vi "Turbulence_3.0_LevelProbe.vi"() -> ()   [LabVIEW 2018]
uses:
  Quantum Composers 9000 Series.lvlib
  LightField Automation.lvclass
  Mercury iXX.lvlib
  Temperature (Read).vi
  Temperature.lvlib
  Open Temperature Device.vi
  Comms Transport Layer.ctl
  Keithley 2600 Series.lvlib
  Channel.ctl
  Open System.vi
  System.lvlib
  Catalogue (Read).vi
panel:
  out "time string":string
  out "Timestamp":string
  out "Log Error":errorcluster
  in  "CLOSE":bool
  in  "RECORD":bool
  in  "Turbulence":T1(tab)
  in  "BIN":u16(ring) items=["1x1", "2x2", "4x4"]
  in  "MODE":u16(ring) items=["Normal", "DIF"]
  in  "Enable":bool
  out "Rate (Hz)":dbl
  out "Neutron Counts":dbl
  in  "Script\nEnd":u32=1 step=1
  in  "Sample Space Pump":bool
  in  "Siphon Pump":bool
  in  "Neutron Shutter":bool
  in  "Manual Script Entry (0)":string
  in  "READY":bool
  out "Power (mW)":dbl format="%_3f"
  out "Tank Pressure 2 (Torr)":string="0.0"
  in  "LIGHTFIELD":bool
  in  "SCRIPTING":bool
  out "Liquid He Level":dbl(slide) min=0.0 max=100.0 step=0.01 scale=0.0..50.0 scale format="%#_2f"
  in  "Top Coil":bool
  in  "Number of Frames":i32=500 min=0 step=1
  in  "On CCD Accumulations":i32=3 min=0 step=1
  out "Tank Pressure 1 (Torr)":string="0.0"
  out "Cell Temp (K)":dbl
  in  "Data folder":path=path "C:/Data"
  out "Cryostat Temp (K)":dbl
  in  "Data Interval (s)":dbl=1.0 min=0.4 max=10.0 step=0.05
  in  "RUN/STOP":bool
  in  "Bottom Coil":bool
  in  "Bottom Coil (mA)":dbl min=-1000.0 max=1000.0 step=1e-05
  in  "Top Coil (mA)":dbl min=-1000.0 max=1000.0 step=1e-05
  in  "Percent Open":i32 min=0 max=100 step=5
  out "Liquid Level":dbl format="%_2f"
  in  "COOLDOWN":bool
  in  "Script\n#":u32=1 step=1
  in  "Kill Switch":bool
  in  "DATA":bool
  out "Scripting \nError":T2
  in  "Shutter Mode":u16(ring) items=["Manual"=1, "XGate"=5]
  in  "Log Pressure":bool
  out "4He Pressure (Torr)":string="-0.1"
  out "3He Pressure (Torr)":string="1"
  out "Temperature Error":errorcluster={"status"=TRUE, "code"=-1073807339, "source"="VISA Read in Mercury iXX.lvlib:Query (Dynamic).vit->Mercury iXX.lvlib:Query (Low Level).vi:10049->Mercury iXX.lvlib:Query.vi:3960048->Mercury iXX.lvlib:Read (Str).vi:5300004->Mercury iXX.lvlib:System.lvlib:Catalogue (Read).vi->Turbulence.vi"}
  out "File I/O Error":errorcluster
  out "4He Gauge Error":errorcluster={"status"=TRUE, "code"=-1073807343, "source"="VISA Open in Turbulence.vi"}
  out "Heater Error":errorcluster={"status"=FALSE, "code"=1073676293, "source"="VISA Read in Keithley 2600 Series.lvlib:Print Number.vi->Keithley 2600 Series.lvlib:Measure.vi->Turbulence.vi"}
  out "Pulse Generator Error":errorcluster
  out "3He Gauge Error":errorcluster={"status"=FALSE, "code"=1073676293, "source"="VISA Read in 3HeClose.vi->Turbulence.vi"}
  out "Relay Errror":errorcluster
  out "Zaber Motor Error":errorcluster
  out "Level Probe Error":errorcluster={"status"=TRUE, "code"=56, "source"="TCP Read in Command.vi->Turbulence.vi"}
  out "LightField Error":errorcluster
  # "Camera Controls"
  # "Temperature Readout"
  # "Pressure Readout"
  # "Liquid He Level"
  # "Automation"
  # "Heater Controls"
  # "Relay Controls"
  # "Needle Valve Control"
  # "Neutron Shutter"
  # "Optical Shutter"
  # "Siphon Pump"
  # "Laser Power Meter"
  # "Sample Space\nPump"
  # "Quartz\nCell"
  # "4"
  # "3psi relief"
  # "4L Tank"
  # "Turbo Pump"
  # "3"
  # "10psi relief"
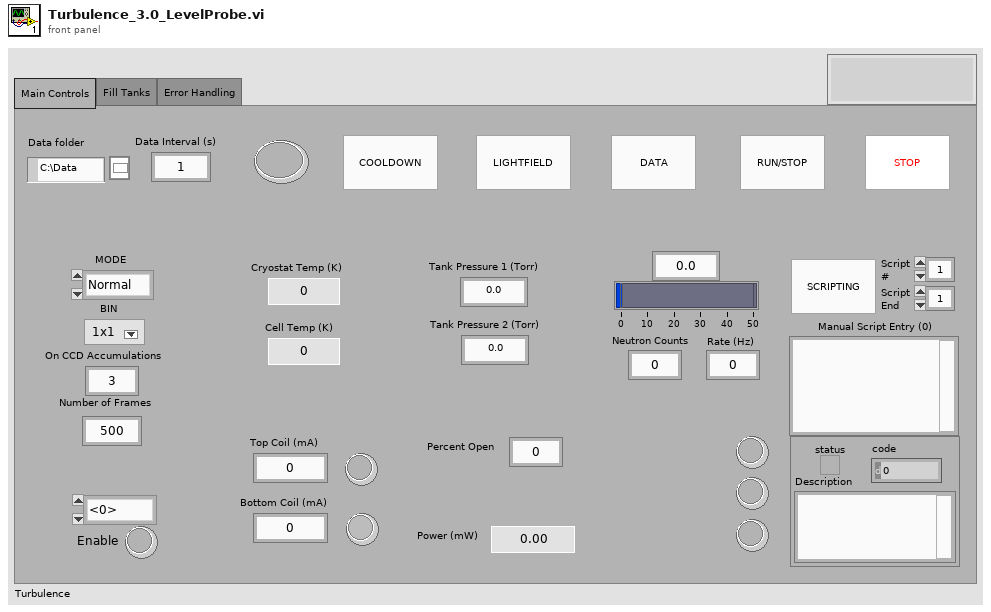
[diagram p1: front panel]
types:
  T1 = enum32{"Main Controls", "Fill Tanks", "Error Handling"}
  T2 = cluster{"status":bool, "code":i32, "Description":string}
  T3 = typedef "Mercury iXX.lvlib/Comms Transport Layer.ctl" = enum16{"Ethernet TCP/IP", "USB", "ISOBus - RS-232", "GPIB"}
  T4 = typedef "Mercury iXX.lvlib/Mercury Reference.ctl" = cluster{"Comms":refnum<visa-resource-name>, "Device ID":string[], "Comms Layer":T3, "Command":string, "Query reference":T5}
  T5 = typedef "Mercury iXX.lvlib/Query Dynamic Reference.ctl" = refnum<vi>
  T6 = enum32{"Current", "Voltage", "IV", "Resistance", "Power"}
  T7 = typedef "Keithley 2600 Series.lvlib/Channel.ctl" = enum32{"Channel A", "Channel B"}
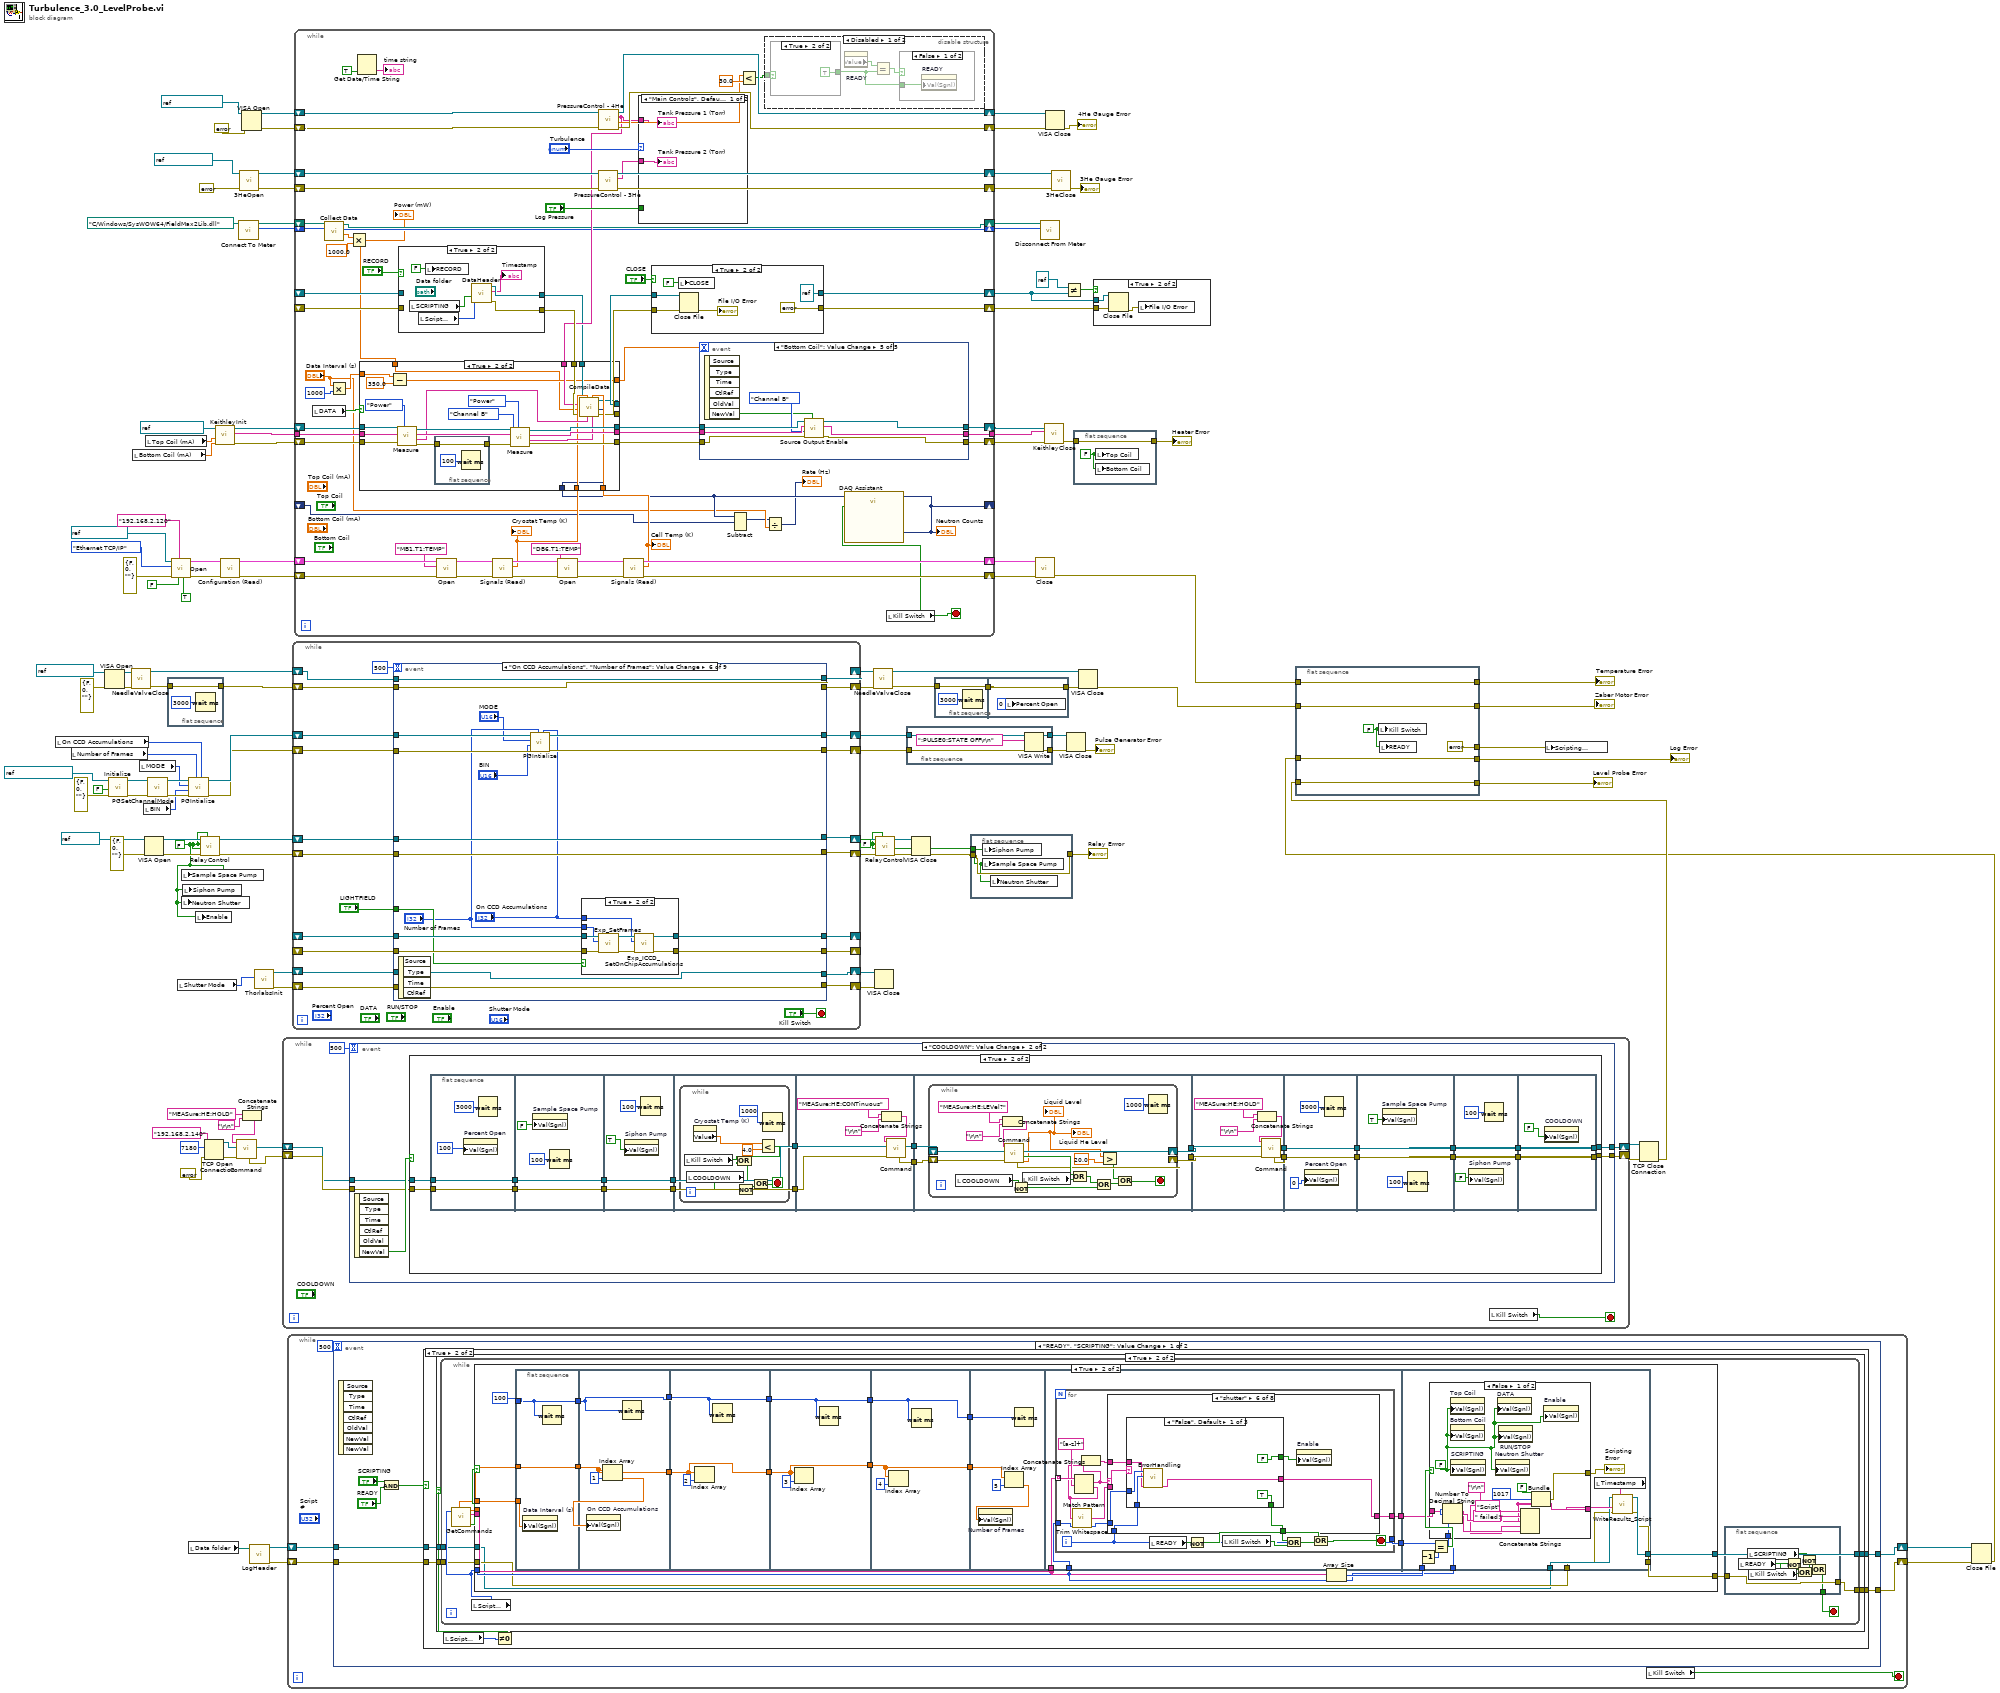
[diagram p0: block diagram]
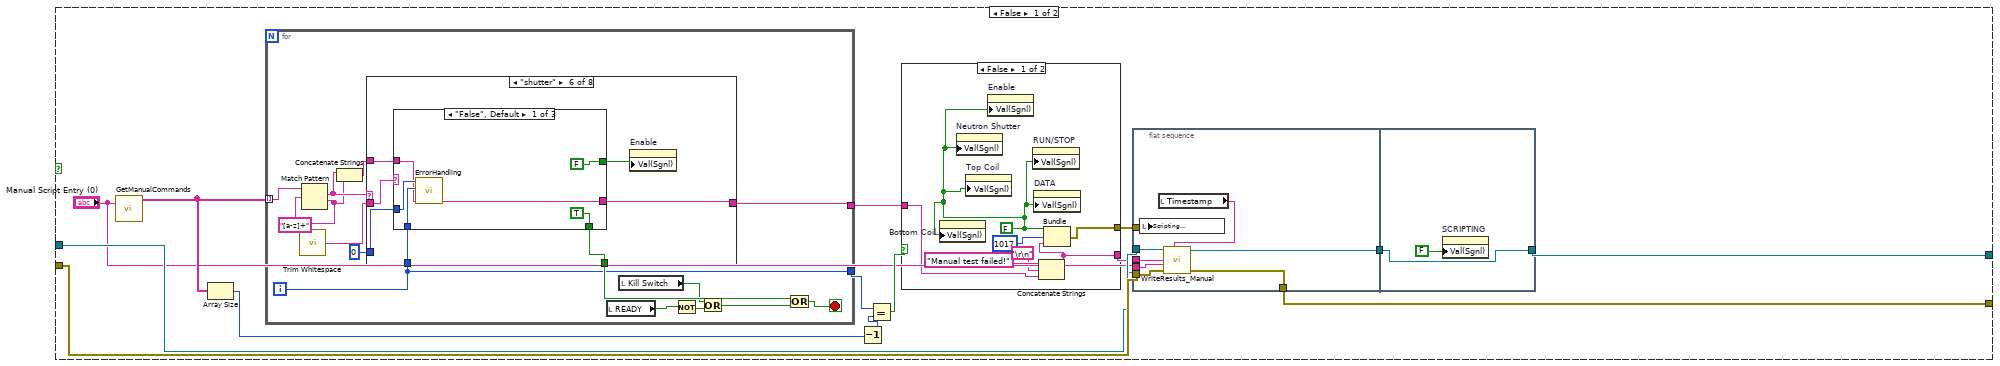
[diagram p3: hidden frame]
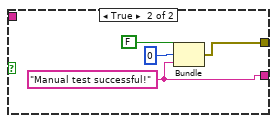
[diagram p4: hidden frame]
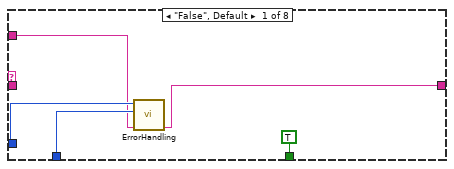
[diagram p5: hidden frame]
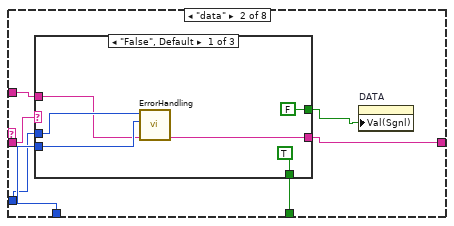
[diagram p6: hidden frame]
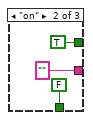
[diagram p7: hidden frame]
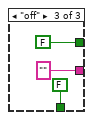
[diagram p8: hidden frame]
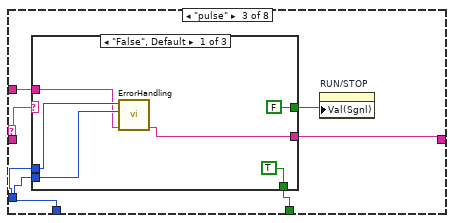
[diagram p9: hidden frame]
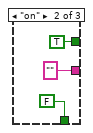
[diagram p10: hidden frame]
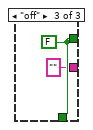
[diagram p11: hidden frame]
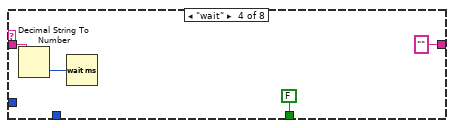
[diagram p12: hidden frame]
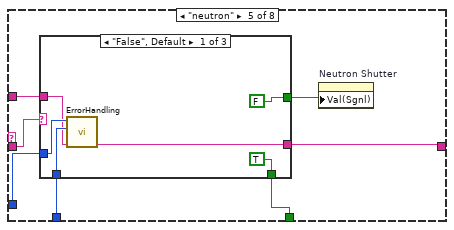
[diagram p13: hidden frame]
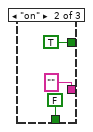
[diagram p14: hidden frame]
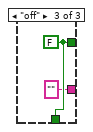
[diagram p15: hidden frame]
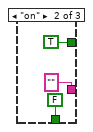
[diagram p16: hidden frame]
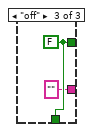
[diagram p17: hidden frame]
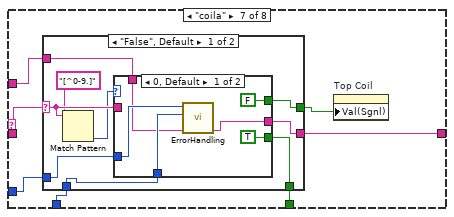
[diagram p18: hidden frame]
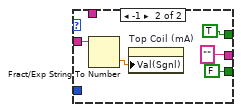
[diagram p19: hidden frame]
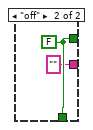
[diagram p20: hidden frame]
diagram:
  w33 = FALSE ("Siphon Pump")
  w17 = FALSE ("Siphon Pump")
  n1 = local read "On CCD Accumulations"() -> (w4:i32)
  n2 = local read "Number of Frames"() -> (w3:i32)
  n3 = VISA Open(error in (no error)=errorcluster {"status"=FALSE, "code"=0, "source"=""}, VISA resource name=refnum<visa-resource-name> "ZaberMotor") -> (VISA resource name=w10:refnum<visa-resource-name>, error out=w11:errorcluster)  [unwired: 3 in]
  n4 = call "Initialize.vi"("error in (no error)"=errorcluster {"status"=FALSE, "code"=0, "source"=""}, "Reset? (T: Yes)"=FALSE, "VISA resource name"=refnum<visa-resource-name> "PulseGenerator" ("Pulse generater (COM3)")) -> ("error out"=w24:errorcluster, "VISA resource name out"=w22:refnum<visa-resource-name>)  [unwired: 7 in]
  n5 = call "NeedleValveClose.vi"("error in (no error)"=w11, "VISA resource name"=w10) -> ("error out"=w12:errorcluster, "VISA resource name out"=w55:refnum<visa-resource-name>)  [unwired: 8 in]
  n6 = local read "Bottom Coil (mA)"() -> (w69:dbl)
  n7 = local read "MODE"() -> (w1:u16)
  n8 = local read "BIN"() -> (w2:u16)
  n9 = VISA Open(error in (no error)=errorcluster {"status"=FALSE, "code"=0, "source"=""} ("error in (no error) 2"), VISA resource name=refnum<visa-resource-name> "Relays" ("Pressure Gauge")) -> (VISA resource name=w94:refnum<visa-resource-name>, error out=w96:errorcluster)  [unwired: 3 in]
  n10 = local read "Top Coil (mA)"() -> (w70:dbl)
  n11 = call "PGSetChannelMode.vi"("error in"=w24, "VISA resource name"=w22) -> ("error out"=w23:errorcluster, "VISA resource name out"=w21:refnum<visa-resource-name>)  [unwired: 8 in]
  n12 = flat-sequence {
    tunnel: w12 -> [w123]
    tunnel: [w123] -> w56
    frame #0 {
      n13 = Wait (ms)(milliseconds to wait=u32 3000) -> ()  [unwired: 1 out]
    }
  }
  n14 = call-poly "Open.vi"("Clear Previous Connections (False)"=TRUE, "ID Query (True)"=FALSE, "IP Address"="192.168.2.120", "error in (no error)"=errorcluster {"status"=FALSE, "code"=0, "source"=""}, "Comms Layer"=Comms_Transport_Layer."Ethernet TCP/IP", "VISA resource name"=refnum<visa-resource-name> "MercuryiTC") -> ("error out"=w115:errorcluster, "Mercury Reference Out"=w116:T4)  [unwired: 1 in, 3 out]
  n15 = local read "Shutter Mode"() -> (w5:u16)
  n16 = local write "Sample Space Pump"(w17) -> ()
  n17 = local write "Neutron Shutter"(w17) -> ()
  n18 = local write "Siphon Pump"(w17) -> ()
  n19 = local read "Data folder"() -> (w31:path)
  n20 = call "PGIntialize.vi"("On CCD Accumulations"=w4, "Number of Frames"=w3, "error in"=w23, "BIN"=w2, "MODE"=w1, "VISA resource name"=w21) -> ("error out"=w120:errorcluster, "VISA resource name out"=w121:refnum<visa-resource-name>)  [unwired: 4 in]
  n21 = local write "Enable"(w17) -> ()
  n22 = call "RelayControl.vi"("Neutron Shutter"=w17, "Error In"=w96, "Sample Space Pump"=w17, "Siphon Pump"=w17, "Relay In"=w94) -> ("Error Out"=w95:errorcluster, "Relay Out"=w93:refnum<visa-resource-name>)  [unwired: 5 in]
  n23 = TCP Open Connection(address="192.168.2.140", remote port or service name=u16 7180, error in (no error)=errorcluster {"status"=FALSE, "code"=0, "source"=""}) -> (connection ID=w80:refnum<k5>, error out=w81:errorcluster)  [unwired: 2 in]
  n24 = call "KeithleyInit.vi"("Bottom Coil (mA)"=w69, "Top Coil (mA)"=w70, "KeithleyVISA In"=refnum<visa-resource-name> "Keithley2614B" ("VISA resource name")) -> ("error out"=w73:errorcluster, "Node Out"=w74:string, "KeithleyVISA Out"=w72:refnum<visa-resource-name>)  [unwired: 6 in]
  n25 = call-poly "Configuration (Read).vi"("error in"=w115, "Mercury Reference In"=w116) -> ("error out"=w111:errorcluster, "Mercury Reference Out"=w112:T4)  [unwired: 6 in, 2 out]
  n26 = call "Connect To Meter.vi"("Location of FieldMax2Lib.dll in"=path "C:/Windows/SysWOW64/FieldMax2Lib.dll") -> ("Meter ID out"=w41:i32, "Location of FieldMax2Lib.dll out"=w40:path)  [unwired: 6 in, 1 out]
  n27 = call "3HeOpen.vi"("error in (no error)"=errorcluster {"status"=FALSE, "code"=0, "source"=""} ("error in (no error) 2"), "VISA resource name"=refnum<visa-resource-name> "3HePressure" ("Pressure Gauge")) -> ("error out"=w98:errorcluster, "VISA resource name out"=w97:refnum<visa-resource-name>)  [unwired: 8 in]
  n28 = VISA Open(error in (no error)=errorcluster {"status"=FALSE, "code"=0, "source"=""} ("error in (no error) 2"), VISA resource name=refnum<visa-resource-name> "TankPressure" ("Pressure Gauge")) -> (VISA resource name=w108:refnum<visa-resource-name>, error out=w109:errorcluster)  [unwired: 3 in]
  n29 = Concatenate Strings("MEASure:HE:HOLD" ("Command"), "\r\n") -> (w82:string)
  n30 = call "Command.vi"("error in"=w81, "connection ID"=w80, "Command"=w82) -> ("connection ID 2"=w79:refnum<k5>, "error out"=w78:errorcluster)  [unwired: 3 in, 4 out]
  n31 = call "LogHeader.vi"("Data folder"=w31) -> ("error out"=w29:errorcluster, "refnum out"=w30:refnum<file>)  [unwired: 9 in]
  n32 = call "ThorlabsInit.vi"("Shutter Mode"=w5) -> ("error out"=w18:errorcluster, "VISA resource name out"=w19:refnum<visa-resource-name>)  [unwired: 9 in]
  n33 = while {
    shift-right: [w125] -> w86
    shift-left: w78 -> [w128]
    shift-right: [w126] -> w85
    shift-left: w79 -> [w127]
    stop <- w130 stop-if-true
    n34 = event shown="[1] \"COOLDOWN\": Value Change" {
      selector: _ -> [_ _]
      dyn-events: _ -> [_ _]
      timeout: 500 -> [_ _]
      tunnel: [w132 w133] -> w126
      tunnel: [w131 w134] -> w125
      tunnel: w128 -> [w131 w136]
      tunnel: w127 -> [w132 w135]
      event Timeout {
        n35 = event-data() -> ()  [unwired: 1 in, 3 out]
      }
      event "COOLDOWN": Value Change {
        n36 = event-data() -> ("NewVal"=w137:bool)  [unwired: 1 in, 5 out]
        n37 = case shown="True" w137 {
          tunnel: [w138 w157] -> w133
          tunnel: [w139 w156] -> w134
          tunnel: w136 -> [w139 w163]
          tunnel: w135 -> [w138 w161]
          frame False {
          }
          frame True {
            n38 = flat-sequence {
              tunnel: w161 -> [w166]
              tunnel: w163 -> [w167]
              tunnel: [w167] -> w149
              tunnel: [w166] -> w148
              tunnel: [w171] -> w147
              tunnel: [w170] -> w145
              tunnel: w149 -> [w171]
              tunnel: w148 -> [w170]
              tunnel: w147 -> [w175]
              tunnel: [w175] -> w146
              tunnel: w145 -> [w174]
              tunnel: [w174] -> w144
              tunnel: [w177] -> w162
              tunnel: w146 -> [w177]
              tunnel: w144 -> [w176]
              tunnel: [w176] -> w160
              tunnel: w162 -> [w190]
              tunnel: w160 -> [w189]
              tunnel: [w188] -> w159
              tunnel: [w187] -> w158
              tunnel: w159 -> [w195]
              tunnel: w158 -> [w194]
              tunnel: [w197] -> w153
              tunnel: [w196] -> w151
              tunnel: w153 -> [w219]
              tunnel: [w216] -> w152
              tunnel: w151 -> [w218]
              tunnel: [w217] -> w150
              tunnel: w152 -> [w226]
              tunnel: [w226] -> w155
              tunnel: w150 -> [w225]
              tunnel: [w225] -> w154
              tunnel: w155 -> [w230]
              tunnel: w154 -> [w229]
              tunnel: [w230] -> w143
              tunnel: [w229] -> w142
              tunnel: w143 -> [w234]
              tunnel: w142 -> [w233]
              tunnel: [w234] -> w141
              tunnel: [w233] -> w140
              tunnel: [w236] -> w156
              tunnel: [w237] -> w157
              tunnel: w141 -> [w237]
              tunnel: w140 -> [w236]
              frame #0 {
                n39 = property on="Percent Open" class="DigNum (strict)"("Val(Sgnl)"=100 ("Percent Open")) -> ()  [unwired: 2 in, 2 out]
                n40 = Wait (ms)(milliseconds to wait=u32 3000) -> ()  [unwired: 1 out]
              }
              frame #1 {
                n41 = property on="Sample Space Pump" class="Bool (strict)"("Val(Sgnl)"=FALSE ("Sample Space Pump")) -> ()  [unwired: 2 in, 2 out]
                n42 = Wait (ms)(milliseconds to wait=u32 100) -> ()  [unwired: 1 out]
              }
              frame #2 {
                n43 = property on="Siphon Pump" class="Bool (strict)"("Val(Sgnl)"=TRUE ("Siphon Pump")) -> ()  [unwired: 2 in, 2 out]
                n44 = Wait (ms)(milliseconds to wait=u32 100) -> ()  [unwired: 1 out]
              }
              frame #3 {
                n45 = while {
                  stop <- w181 stop-if-true
                  n46 = local read "Kill Switch"() -> (w184:bool)
                  n47 = local read "COOLDOWN"() -> (w179:bool)
                  n48 = property on="Cryostat Temp (K)" class="DigNum (strict)"() -> ("Value"=w186:dbl)  [unwired: 2 in, 2 out]
                  n49 = Not(x=w179) -> (.not. x?=w178:bool)
                  n50 = Less?(x=w186, y=4.0) -> (x < y?=w183:bool)
                  n51 = Or(x=w184, y=w183) -> (x .or. y?=w180:bool)
                  n52 = Or(x=w180, y=w178) -> (x .or. y?=w181:bool)
                  n53 = Wait (ms)(milliseconds to wait=u32 1000) -> ()  [unwired: 1 out]
                }
              }
              frame #4 {
                n54 = Concatenate Strings("MEASure:HE:CONTinuous" ("Command"), "\r\n") -> (w191:string)
                n55 = call "Command.vi"("error in"=w190, "connection ID"=w189, "Command"=w191) -> ("connection ID 2"=w187:refnum<k5>, "error out"=w188:errorcluster)  [unwired: 3 in, 4 out]
              }
              frame #5 {
                n56 = while {
                  shift-right: [w213] -> w197
                  shift-left: w194 -> [w214]
                  shift-right: [w207] -> w196
                  shift-left: w195 -> [w215]
                  stop <- w202 stop-if-true
                  n57 = local read "COOLDOWN"() -> (w199:bool)
                  n58 = Concatenate Strings("MEASure:HE:LEVel?" ("Command"), "\r\n") -> (w212:string)
                  n59 = call "Command.vi"("error in"=w215, "connection ID"=w214, "Command"=w212) -> ("Dbl_out"=w205:dbl, "Error"=w208:bool, "connection ID 2"=w213:refnum<k5>, "error out"=w207:errorcluster)  [unwired: 3 in, 2 out]
                  "Liquid He Level" <- w205
                  "Liquid Level" <- w205
                  n60 = Not(x=w199) -> (.not. x?=w198:bool)
                  n61 = local read "Kill Switch"() -> (w209:bool)
                  n62 = Or(x=w208, y=w209) -> (x .or. y?=w201:bool)
                  n63 = Or(x=w201, y=w198) -> (x .or. y?=w200:bool)
                  n64 = Greater?(x=w205, y=20.0) -> (0:w203:bool)
                  n65 = Or(x=w203, y=w200) -> (x .or. y?=w202:bool)
                  n66 = Wait (ms)(milliseconds to wait=u32 1000) -> ()  [unwired: 1 out]
                }
              }
              frame #6 {
                n67 = Concatenate Strings("MEASure:HE:HOLD" ("Command"), "\r\n") -> (w220:string)
                n68 = call "Command.vi"("error in"=w218, "connection ID"=w219, "Command"=w220) -> ("connection ID 2"=w216:refnum<k5>, "error out"=w217:errorcluster)  [unwired: 3 in, 4 out]
              }
              frame #7 {
                n69 = property on="Percent Open" class="DigNum (strict)"("Val(Sgnl)"=0 ("Percent Open")) -> ()  [unwired: 2 in, 2 out]
                n70 = Wait (ms)(milliseconds to wait=u32 3000) -> ()  [unwired: 1 out]
              }
              frame #8 {
                n71 = property on="Sample Space Pump" class="Bool (strict)"("Val(Sgnl)"=TRUE ("Sample Space Pump")) -> ()  [unwired: 2 in, 2 out]
                n72 = Wait (ms)(milliseconds to wait=u32 100) -> ()  [unwired: 1 out]
              }
              frame #9 {
                n73 = property on="Siphon Pump" class="Bool (strict)"("Val(Sgnl)"=FALSE ("Siphon Pump")) -> ()  [unwired: 2 in, 2 out]
                n74 = Wait (ms)(milliseconds to wait=u32 100) -> ()  [unwired: 1 out]
              }
              frame #10 {
                n75 = property on="COOLDOWN" class="Bool (strict)"("Val(Sgnl)"=FALSE ("COOLDOWN")) -> ()  [unwired: 2 in, 2 out]
              }
            }
          }
        }
      }
    }
    n76 = local read "Kill Switch"() -> (w130:bool)
  }
  n77 = while {
    shift-right: [w239] -> w28
    shift-left: w30 -> [w240]
    shift-right: [w238] -> w27
    shift-left: w29 -> [w241]
    stop <- w243 stop-if-true
    n78 = event shown="[0] \"READY\", \"SCRIPTING\": Value Change" {
      selector: _ -> [_ _]
      dyn-events: _ -> [_ _]
      timeout: 500 -> [_ _]
      tunnel: w241 -> [w247 w727]
      tunnel: w240 -> [w248 w728]
      tunnel: [w246 w728] -> w239
      tunnel: [w245 w727] -> w238
      event "READY", "SCRIPTING": Value Change {
        n79 = event-data() -> ()  [unwired: 1 in, 7 out]
        n80 = And(x="SCRIPTING", y="READY") -> (x .and. y?=w244:bool)
        n81 = case shown="True" w244 {
          tunnel: w248 -> [w252 w256]
          tunnel: w247 -> [w251 w255]
          tunnel: [w252 w253] -> w246
          tunnel: [w251 w254] -> w245
          frame False {
          }
          frame True {
            n82 = local read "Script\n#"() -> (w258:u32)
            n83 = Not Equal To 0?(x=w258) -> (x != 0?=w257:bool)
            n84 = case shown="True" w257 {
              tunnel: w256 -> [w264 w451]
              tunnel: w255 -> [w265 w452]
              tunnel: [w259 w449] -> w254
              tunnel: [w260 w450] -> w253
              frame False {
                n85 = call "GetManualCommands.vi"("Manual Script Entry (0)"="Manual Script Entry (0)") -> ("Commands"=w272:string[])  [unwired: 10 in]
                n86 = Array Size(array=w272) -> (size(s)=w268:i32)
                n87 = for {
                  tunnel: w272 -> [w307] mode=indexing
                  tunnel: [w298] -> w271
                  tunnel: [w297] -> w266
                  i -> [w298]
                  stop <- w304 stop-if-true
                  n88 = Match Pattern(string=w307, regular expression="[a-z]+") -> (match substring=w296:string, after substring=w295:string)  [unwired: 1 in, 2 out]
                  n89 = call "Trim Whitespace.vi"("string"=w295) -> ("trimmed string"=w306:string)  [unwired: 1 in]
                  n90 = Concatenate Strings(w296, w295) -> (w294:string)
                  n91 = case shown="\"shutter\"" w296 {
                    tunnel: w306 -> [_ w320 w339 w354 w361 w379 w397 w426]
                    tunnel: [TRUE ("Top Coil") w319 w336 FALSE ("Top Coil") w358 w376 w396 w425] -> w303
                    tunnel: w298 -> [w312 w318 w338 _ w360 w378 w395 w424]
                    tunnel: u32 0 ("Script Number") -> [w311 w317 w337 _ w359 w377 w394 w423]
                    tunnel: [w310 w315 w334 "" ("Error String") w356 w375 w392 w421] -> w297
                    tunnel: w294 -> [w309 w314 w333 _ w355 w374 w391 w420]
                    frame "False", Default {
                      n92 = call "ErrorHandling.vi"("Bad Command"=w309, "Line #"=w312, "Script #"=w311) -> ("Error String"=w310:string)  [unwired: 8 in]
                    }
                    frame "data" {
                      n93 = case shown="\"False\", Default" w320 {
                        tunnel: [FALSE ("DATA") TRUE ("DATA") FALSE ("DATA")] -> w316
                        tunnel: [TRUE ("Top Coil") FALSE ("Top Coil") FALSE ("Top Coil")] -> w319
                        tunnel: w318 -> [w323 _ _]
                        tunnel: w317 -> [w324 _ _]
                        tunnel: [w322 "" ("Error String") "" ("Error String")] -> w315
                        tunnel: w314 -> [w321 _ _]
                        frame "False", Default {
                          n94 = call "ErrorHandling.vi"("Bad Command"=w321, "Line #"=w323, "Script #"=w324) -> ("Error String"=w322:string)  [unwired: 8 in]
                        }
                        frame "on" {
                        }
                        frame "off" {
                        }
                      }
                      n95 = property on="DATA" class="Bool (strict)"("Val(Sgnl)"=w316) -> ()  [unwired: 2 in, 2 out]
                    }
                    frame "pulse" {
                      n96 = case shown="\"False\", Default" w339 {
                        tunnel: [FALSE ("Top Coil") TRUE ("Top Coil") w350] -> w335
                        tunnel: [TRUE FALSE w350] -> w336
                        tunnel: w338 -> [w343 _ _]
                        tunnel: w337 -> [w342 _ _]
                        tunnel: [w341 "" ""] -> w334
                        tunnel: w333 -> [w340 _ _]
                        frame "False", Default {
                          n97 = call "ErrorHandling.vi"("Bad Command"=w340, "Line #"=w343, "Script #"=w342) -> ("Error String"=w341:string)  [unwired: 8 in]
                        }
                        frame "on" {
                        }
                        frame "off" {
                          w350 = FALSE ("Top Coil")
                        }
                      }
                      n98 = property on="RUN/STOP" class="Bool (strict)"("Val(Sgnl)"=w335) -> ()  [unwired: 2 in, 2 out]
                    }
                    frame "wait" {
                      n99 = Decimal String To Number(string=w354) -> (number=w353:i32)  [unwired: 2 in, 1 out]
                      n100 = Wait (ms)(milliseconds to wait=w353) -> ()  [unwired: 1 out]
                    }
                    frame "neutron" {
                      n101 = case shown="\"False\", Default" w361 {
                        tunnel: w360 -> [w367 _ _]
                        tunnel: w359 -> [w366 _ _]
                        tunnel: [TRUE ("Top Coil") FALSE ("Top Coil") w372] -> w358
                        tunnel: [FALSE ("Neutron Shutter") TRUE ("Neutron Shutter") w372] -> w357
                        tunnel: [w363 "" ("Error String") "" ("Error String")] -> w356
                        tunnel: w355 -> [w362 _ _]
                        frame "False", Default {
                          n102 = call "ErrorHandling.vi"("Bad Command"=w362, "Line #"=w367, "Script #"=w366) -> ("Error String"=w363:string)  [unwired: 8 in]
                        }
                        frame "on" {
                        }
                        frame "off" {
                          w372 = FALSE ("Neutron Shutter")
                        }
                      }
                      n103 = property on="Neutron Shutter" class="Bool (strict)"("Val(Sgnl)"=w357) -> ()  [unwired: 2 in, 2 out]
                    }
                    frame "shutter" {
                      n104 = case shown="\"False\", Default" w379 {
                        tunnel: w378 -> [w385 _ _]
                        tunnel: w377 -> [w384 _ _]
                        tunnel: [TRUE ("Top Coil") FALSE ("Top Coil") w390] -> w376
                        tunnel: [FALSE ("Neutron Shutter") TRUE ("Neutron Shutter") w390] -> w373
                        tunnel: [w381 "" ("Error String") "" ("Error String")] -> w375
                        tunnel: w374 -> [w380 _ _]
                        frame "False", Default {
                          n105 = call "ErrorHandling.vi"("Bad Command"=w380, "Line #"=w385, "Script #"=w384) -> ("Error String"=w381:string)  [unwired: 8 in]
                        }
                        frame "on" {
                        }
                        frame "off" {
                          w390 = FALSE ("Neutron Shutter")
                        }
                      }
                      n106 = property on="Enable" class="Bool (strict)"("Val(Sgnl)"=w373) -> ()  [unwired: 2 in, 2 out]
                    }
                    frame "coila" {
                      n107 = case shown="\"False\", Default" w397 {
                        selector: w397 -> [w404 _]
                        tunnel: [w406 w419] -> w393
                        tunnel: [w405 w419] -> w396
                        tunnel: w395 -> [w401 _]
                        tunnel: w394 -> [w400 _]
                        tunnel: [w399 "" ("Error String")] -> w392
                        tunnel: w391 -> [w398 _]
                        frame "False", Default {
                          n108 = Match Pattern(string=w404, regular expression="[^0-9.]") -> (offset past match=w402:i32)  [unwired: 1 in, 3 out]
                          n109 = case shown="0, Default" w402 {
                            tunnel: [FALSE ("Top Coil") TRUE ("Top Coil")] -> w406
                            tunnel: [TRUE FALSE] -> w405
                            tunnel: w404 -> [_ w415]
                            tunnel: w401 -> [w410 _]
                            tunnel: w400 -> [w409 _]
                            tunnel: [w408 ""] -> w399
                            tunnel: w398 -> [w407 _]
                            frame 0, Default {
                              n110 = call "ErrorHandling.vi"("Bad Command"=w407, "Line #"=w410, "Script #"=w409) -> ("Error String"=w408:string)  [unwired: 8 in]
                            }
                            frame -1 {
                              n111 = Fract/Exp String To Number(string=w415) -> (number=w414:dbl)  [unwired: 3 in, 1 out]
                              n112 = property on="Top Coil (mA)" class="DigNum (strict)"("Val(Sgnl)"=w414) -> ()  [unwired: 2 in, 2 out]
                            }
                          }
                        }
                        frame "off" {
                          w419 = FALSE ("Top Coil")
                        }
                      }
                      n113 = property on="Top Coil" class="Bool (strict)"("Val(Sgnl)"=w393) -> ()  [unwired: 2 in, 2 out]
                    }
                    frame "coilb" {
                      n114 = case shown="\"False\", Default" w426 {
                        selector: w426 -> [w433 _]
                        tunnel: [w432 w448] -> w422
                        tunnel: [w431 w448] -> w425
                        tunnel: w424 -> [w430 _]
                        tunnel: w423 -> [w429 _]
                        tunnel: [w428 ""] -> w421
                        tunnel: w420 -> [w427 _]
                        frame "False", Default {
                          n115 = Match Pattern(string=w433, regular expression="[^0-9.]") -> (offset past match=w434:i32)  [unwired: 1 in, 3 out]
                          n116 = case shown="0, Default" w434 {
                            tunnel: w433 -> [_ w446]
                            tunnel: [FALSE TRUE] -> w432
                            tunnel: [TRUE FALSE] -> w431
                            tunnel: w430 -> [w439 _]
                            tunnel: w429 -> [w438 _]
                            tunnel: [w437 ""] -> w428
                            tunnel: w427 -> [w436 _]
                            frame 0, Default {
                              n117 = call "ErrorHandling.vi"("Bad Command"=w436, "Line #"=w439, "Script #"=w438) -> ("Error String"=w437:string)  [unwired: 8 in]
                            }
                            frame -1 {
                              n118 = Fract/Exp String To Number(string=w446) -> (number=w443:dbl)  [unwired: 3 in, 1 out]
                              n119 = property on="Bottom Coil (mA)" class="DigNum (strict)"("Val(Sgnl)"=w443) -> ()  [unwired: 2 in, 2 out]
                            }
                          }
                        }
                        frame "off" {
                          w448 = FALSE
                        }
                      }
                      n120 = property on="Bottom Coil" class="Bool (strict)"("Val(Sgnl)"=w422) -> ()  [unwired: 2 in, 2 out]
                    }
                  }
                  n121 = local read "READY"() -> (w299:bool)
                  n122 = local read "Kill Switch"() -> (w300:bool)
                  n123 = Not(x=w299) -> (.not. x?=w302:bool)
                  n124 = Or(x=w300, y=w302) -> (x .or. y?=w301:bool)
                  n125 = Or(x=w303, y=w301) -> (x .or. y?=w304:bool)
                }
                n126 = Decrement(x=w268) -> (x-1=w270:i32)
                n127 = Equal?(x=w271, y=w270) -> (x = y?=w269:bool)
                n128 = case shown="False" w269 {
                  tunnel: [w288 w291] -> w267
                  tunnel: w266 -> [w286 _]
                  tunnel: [w284 w290] -> w262
                  frame False {
                    w283 = FALSE ("status")
                    n129 = property on="Bottom Coil" class="Bool (strict)"("Val(Sgnl)"=w283) -> ()  [unwired: 2 in, 2 out]
                    n130 = property on="Neutron Shutter" class="Bool (strict)"("Val(Sgnl)"=w283) -> ()  [unwired: 2 in, 2 out]
                    n131 = property on="Top Coil" class="Bool (strict)"("Val(Sgnl)"=w283) -> ()  [unwired: 2 in, 2 out]
                    n132 = property on="Enable" class="Bool (strict)"("Val(Sgnl)"=w283) -> ()  [unwired: 2 in, 2 out]
                    n133 = property on="RUN/STOP" class="Bool (strict)"("Val(Sgnl)"=w283) -> ()  [unwired: 2 in, 2 out]
                    n134 = property on="DATA" class="Bool (strict)"("Val(Sgnl)"=w283) -> ()  [unwired: 2 in, 2 out]
                    n135 = Concatenate Strings("Manual test failed!" ("Description"), "\r\n", w286) -> (w284:string)
                    n136 = Bundle("status"=w283, "code"=1017, w284) -> (w288:cluster{"status":bool, "code":i32, string})  [unwired: 1 in]
                  }
                  frame True {
                    w290 = "Manual test successful!" ("Description")
                    n137 = Bundle("status"=FALSE, "code"=0, "Description"=w290) -> (w291:T2)  [unwired: 1 in]
                  }
                }
                n138 = flat-sequence {
                  tunnel: w267 -> [w280]
                  tunnel: w265 -> [w276]
                  tunnel: w264 -> [w279]
                  tunnel: "Manual Script Entry (0)" -> [w278]
                  tunnel: w262 -> [w277]
                  tunnel: [w275] -> w261
                  tunnel: [w274] -> w259
                  tunnel: w261 -> [w282]
                  tunnel: [w282] -> w260
                  frame #0 {
                    n139 = local write "Scripting \nError"(w280) -> ()
                    n140 = local read "Timestamp"() -> (w273:string)
                    n141 = call "WriteResults_Manual.vi"("Timestamp"=w273, "error in"=w276, "Result"=w277, "Commands"=w278, "refnum in"=w279) -> ("error out"=w274:errorcluster, "refnum out"=w275:refnum<file>)  [unwired: 5 in]
                  }
                  frame #1 {
                    n142 = property on="SCRIPTING" class="Bool (strict)"("Val(Sgnl)"=FALSE ("Value (Signaling)")) -> ()  [unwired: 2 in, 2 out]
                  }
                }
              }
              frame True {
                n143 = while {
                  tunnel: w452 -> [w458]
                  tunnel: w451 -> [w457]
                  tunnel: [w456] -> w450
                  tunnel: [w454] -> w449
                  stop <- w453 stop-if-true
                  n144 = local read "Script\n#"() -> (w460:u32)
                  n145 = call "GetCommands.vi"("Script Number"=w460) -> ("Script Exists"=w461:bool, "Commands"=w462:string[], "Camera Settings"=w463:dbl[], "Data Interval (s)"=w459:dbl)  [unwired: 5 in]
                  n146 = case shown="True" w461 {
                    tunnel: w463 -> [_ w500]
                    tunnel: w462 -> [_ w498]
                    tunnel: w460 -> [w483 w496]
                    tunnel: w459 -> [_ w495]
                    tunnel: w458 -> [w477 w493]
                    tunnel: w457 -> [w478 w492]
                    tunnel: [w476 w491] -> w456
                    tunnel: [w475 w490] -> w455
                    frame False {
                      n147 = Number To Decimal String(number=w483) -> (decimal integer string=w482:string)  [unwired: 1 in]
                      n148 = Concatenate Strings("Script" ("string"), w482, " does not exist." ("string")) -> (w479:string)
                      n149 = Bundle("status"=FALSE, "code"=1017, w479) -> (w484:cluster{"status":bool, "code":i32, string})  [unwired: 1 in]
                      n150 = Get Date/Time In Seconds() -> (seconds since 1Jan1904=w474:timestamp)
                      n151 = Format Date/Time String(time format string (%c)="%H:%M:%S", seconds (now)=w474) -> (date/time string=w472:string)  [unwired: 1 in]
                      n152 = local write "Scripting \nError"(w484) -> ()
                      n153 = call "WriteResults_Script.vi"("Timestamp"=w472, "error in"=w477, "Result"=w479, "refnum in"=w478) -> ("error out"=w475:errorcluster, "refnum out"=w476:refnum<file>)  [unwired: 6 in]
                      n154 = property on="SCRIPTING" class="Bool (strict)"("Val(Sgnl)"=FALSE ("Value (Signaling)")) -> ()  [unwired: 2 in, 2 out]
                    }
                    frame True {
                      n155 = flat-sequence {
                        tunnel: u32 100 ("milliseconds to wait") -> [w511]
                        tunnel: w500 -> [w512]
                        tunnel: [w512] -> w489
                        tunnel: [w511] -> w488
                        tunnel: w495 -> [w510]
                        tunnel: w489 -> [w515]
                        tunnel: [w515] -> w509
                        tunnel: w488 -> [w514]
                        tunnel: [w514] -> w508
                        tunnel: w509 -> [w518]
                        tunnel: [w518] -> w507
                        tunnel: w508 -> [w517]
                        tunnel: [w517] -> w506
                        tunnel: w507 -> [w521]
                        tunnel: [w521] -> w505
                        tunnel: w506 -> [w520]
                        tunnel: [w520] -> w504
                        tunnel: w505 -> [w524]
                        tunnel: [w524] -> w503
                        tunnel: w504 -> [w523]
                        tunnel: [w523] -> w502
                        tunnel: w503 -> [w528]
                        tunnel: w502 -> [w527]
                        tunnel: w498 -> [w533]
                        tunnel: w496 -> [w532]
                        tunnel: [w531] -> w501
                        tunnel: [w530] -> w494
                        tunnel: w497 -> [w699]
                        tunnel: w501 -> [w700]
                        tunnel: w496 -> [w689]
                        tunnel: w494 -> [w696]
                        tunnel: w493 -> [w693]
                        tunnel: w492 -> [w694]
                        tunnel: [w692] -> w491
                        tunnel: [w691] -> w490
                        frame #0 {
                          n156 = property on="Data Interval (s)" class="DigNum (strict)"("Val(Sgnl)"=w510) -> ()  [unwired: 2 in, 2 out]
                          n157 = Wait (ms)(milliseconds to wait=w511) -> ()  [unwired: 1 out]
                        }
                        frame #1 {
                          n158 = Index Array(array=w515, index=1) -> (element=w513:dbl)
                          n159 = property on="On CCD Accumulations" class="DigNum (strict)"("Val(Sgnl)"=w513) -> ()  [unwired: 2 in, 2 out]
                          n160 = Wait (ms)(milliseconds to wait=w514) -> ()  [unwired: 1 out]
                        }
                        frame #2 {
                          n161 = Index Array(array=w518, index=2) -> ()  [unwired: 1 out]
                          n162 = Wait (ms)(milliseconds to wait=w517) -> ()  [unwired: 1 out]
                        }
                        frame #3 {
                          n163 = Index Array(array=w521, index=3) -> ()  [unwired: 1 out]
                          n164 = Wait (ms)(milliseconds to wait=w520) -> ()  [unwired: 1 out]
                        }
                        frame #4 {
                          n165 = Index Array(array=w524, index=4) -> ()  [unwired: 1 out]
                          n166 = Wait (ms)(milliseconds to wait=w523) -> ()  [unwired: 1 out]
                        }
                        frame #5 {
                          n167 = Index Array(array=w528, index=5) -> (element=w526:dbl)
                          n168 = property on="Number of Frames" class="DigNum (strict)"("Val(Sgnl)"=w526) -> ()  [unwired: 2 in, 2 out]
                          n169 = Wait (ms)(milliseconds to wait=w527) -> ()  [unwired: 1 out]
                        }
                        frame #6 {
                          n170 = for {
                            tunnel: w533 -> [w548] mode=indexing
                            tunnel: w532 -> [w545]
                            tunnel: [w538] -> w531
                            tunnel: [w537] -> w530
                            i -> [w538]
                            stop <- w541 stop-if-true
                            n171 = Match Pattern(string=w548, regular expression="[a-z]+") -> (match substring=w536:string, after substring=w535:string)  [unwired: 1 in, 2 out]
                            n172 = call "Trim Whitespace.vi"("string"=w535) -> ("trimmed string"=w546:string)  [unwired: 1 in]
                            n173 = Concatenate Strings(w536, w535) -> (w534:string)
                            n174 = case shown="\"shutter\"" w536 {
                              tunnel: w546 -> [_ w560 w579 w594 w601 w619 w637 w666]
                              tunnel: [TRUE ("Top Coil") w559 w576 FALSE ("Top Coil") w598 w616 w636 w665] -> w544
                              tunnel: w538 -> [w552 w558 w578 _ w600 w618 w635 w664]
                              tunnel: w545 -> [w551 w557 w577 _ w599 w617 w634 w663]
                              tunnel: [w549 w555 w574 "" ("Error String") w596 w615 w632 w661] -> w537
                              tunnel: w534 -> [w550 w554 w573 _ w595 w614 w631 w660]
                              frame "False", Default {
                                n175 = call "ErrorHandling.vi"("Bad Command"=w550, "Line #"=w552, "Script #"=w551) -> ("Error String"=w549:string)  [unwired: 8 in]
                              }
                              frame "data" {
                                n176 = case shown="\"False\", Default" w560 {
                                tunnel: [FALSE ("DATA") TRUE ("DATA") FALSE ("DATA")] -> w556
                                tunnel: [TRUE ("Top Coil") FALSE ("Top Coil") FALSE ("Top Coil")] -> w559
                                tunnel: w558 -> [w563 _ _]
                                tunnel: w557 -> [w564 _ _]
                                tunnel: [w562 "" ""] -> w555
                                tunnel: w554 -> [w561 _ _]
                                frame "False", Default {
                                n177 = call "ErrorHandling.vi"("Bad Command"=w561, "Line #"=w563, "Script #"=w564) -> ("Error String"=w562:string)  [unwired: 8 in]
                                }
                                frame "on" {
                                }
                                frame "off" {
                                }
                                }
                                n178 = property on="DATA" class="Bool (strict)"("Val(Sgnl)"=w556) -> ()  [unwired: 2 in, 2 out]
                              }
                              frame "pulse" {
                                n179 = case shown="\"False\", Default" w579 {
                                tunnel: [FALSE ("Top Coil") TRUE ("Top Coil") w590] -> w575
                                tunnel: [TRUE FALSE w590] -> w576
                                tunnel: w578 -> [w583 _ _]
                                tunnel: w577 -> [w582 _ _]
                                tunnel: [w581 "" ("Error String") ""] -> w574
                                tunnel: w573 -> [w580 _ _]
                                frame "False", Default {
                                n180 = call "ErrorHandling.vi"("Bad Command"=w580, "Line #"=w583, "Script #"=w582) -> ("Error String"=w581:string)  [unwired: 8 in]
                                }
                                frame "on" {
                                }
                                frame "off" {
                                w590 = FALSE ("Top Coil")
                                }
                                }
                                n181 = property on="RUN/STOP" class="Bool (strict)"("Val(Sgnl)"=w575) -> ()  [unwired: 2 in, 2 out]
                              }
                              frame "wait" {
                                n182 = Decimal String To Number(string=w594) -> (number=w593:i32)  [unwired: 2 in, 1 out]
                                n183 = Wait (ms)(milliseconds to wait=w593) -> ()  [unwired: 1 out]
                              }
                              frame "neutron" {
                                n184 = case shown="\"False\", Default" w601 {
                                tunnel: w600 -> [w607 _ _]
                                tunnel: w599 -> [w606 _ _]
                                tunnel: [TRUE ("Top Coil") FALSE ("Top Coil") w612] -> w598
                                tunnel: [FALSE ("Neutron Shutter") TRUE ("Neutron Shutter") w612] -> w597
                                tunnel: [w603 "" ""] -> w596
                                tunnel: w595 -> [w602 _ _]
                                frame "False", Default {
                                n185 = call "ErrorHandling.vi"("Bad Command"=w602, "Line #"=w607, "Script #"=w606) -> ("Error String"=w603:string)  [unwired: 8 in]
                                }
                                frame "on" {
                                }
                                frame "off" {
                                w612 = FALSE ("Neutron Shutter")
                                }
                                }
                                n186 = property on="Neutron Shutter" class="Bool (strict)"("Val(Sgnl)"=w597) -> ()  [unwired: 2 in, 2 out]
                              }
                              frame "shutter" {
                                n187 = case shown="\"False\", Default" w619 {
                                tunnel: w618 -> [w625 _ _]
                                tunnel: w617 -> [w624 _ _]
                                tunnel: [TRUE ("Top Coil") FALSE ("Top Coil") w630] -> w616
                                tunnel: [FALSE ("Neutron Shutter") TRUE ("Neutron Shutter") w630] -> w613
                                tunnel: [w621 "" ""] -> w615
                                tunnel: w614 -> [w620 _ _]
                                frame "False", Default {
                                n188 = call "ErrorHandling.vi"("Bad Command"=w620, "Line #"=w625, "Script #"=w624) -> ("Error String"=w621:string)  [unwired: 8 in]
                                }
                                frame "on" {
                                }
                                frame "off" {
                                w630 = FALSE ("Neutron Shutter")
                                }
                                }
                                n189 = property on="Enable" class="Bool (strict)"("Val(Sgnl)"=w613) -> ()  [unwired: 2 in, 2 out]
                              }
                              frame "coila" {
                                n190 = case shown="\"False\", Default" w637 {
                                selector: w637 -> [w644 _]
                                tunnel: [w646 w659] -> w633
                                tunnel: [w645 w659] -> w636
                                tunnel: w635 -> [w641 _]
                                tunnel: w634 -> [w640 _]
                                tunnel: [w639 ""] -> w632
                                tunnel: w631 -> [w638 _]
                                frame "False", Default {
                                n191 = Match Pattern(string=w644, regular expression="[^0-9.]") -> (offset past match=w642:i32)  [unwired: 1 in, 3 out]
                                n192 = case shown="-1" w642 {
                                tunnel: [FALSE ("Top Coil") TRUE ("Top Coil")] -> w646
                                tunnel: [TRUE FALSE] -> w645
                                tunnel: w644 -> [_ w655]
                                tunnel: w641 -> [w650 _]
                                tunnel: w640 -> [w649 _]
                                tunnel: [w648 ""] -> w639
                                tunnel: w638 -> [w647 _]
                                frame 0, Default {
                                n193 = call "ErrorHandling.vi"("Bad Command"=w647, "Line #"=w650, "Script #"=w649) -> ("Error String"=w648:string)  [unwired: 8 in]
                                }
                                frame -1 {
                                n194 = Fract/Exp String To Number(string=w655) -> (number=w654:dbl)  [unwired: 3 in, 1 out]
                                n195 = property on="Top Coil (mA)" class="DigNum (strict)"("Val(Sgnl)"=w654) -> ()  [unwired: 2 in, 2 out]
                                }
                                }
                                }
                                frame "off" {
                                w659 = FALSE ("Top Coil")
                                }
                                }
                                n196 = property on="Top Coil" class="Bool (strict)"("Val(Sgnl)"=w633) -> ()  [unwired: 2 in, 2 out]
                              }
                              frame "coilb" {
                                n197 = case shown="\"off\"" w666 {
                                selector: w666 -> [w673 _]
                                tunnel: [w672 w688] -> w662
                                tunnel: [w671 w688] -> w665
                                tunnel: w664 -> [w670 _]
                                tunnel: w663 -> [w669 _]
                                tunnel: [w668 "" ("Error String")] -> w661
                                tunnel: w660 -> [w667 _]
                                frame "False", Default {
                                n198 = Match Pattern(string=w673, regular expression="[^0-9.]") -> (offset past match=w674:i32)  [unwired: 1 in, 3 out]
                                n199 = case shown="-1" w674 {
                                tunnel: w673 -> [_ w686]
                                tunnel: [FALSE TRUE] -> w672
                                tunnel: [TRUE FALSE] -> w671
                                tunnel: w670 -> [w679 _]
                                tunnel: w669 -> [w678 _]
                                tunnel: [w677 ""] -> w668
                                tunnel: w667 -> [w676 _]
                                frame 0, Default {
                                n200 = call "ErrorHandling.vi"("Bad Command"=w676, "Line #"=w679, "Script #"=w678) -> ("Error String"=w677:string)  [unwired: 8 in]
                                }
                                frame -1 {
                                n201 = Fract/Exp String To Number(string=w686) -> (number=w683:dbl)  [unwired: 3 in, 1 out]
                                n202 = property on="Bottom Coil (mA)" class="DigNum (strict)"("Val(Sgnl)"=w683) -> ()  [unwired: 2 in, 2 out]
                                }
                                }
                                }
                                frame "off" {
                                w688 = FALSE
                                }
                                }
                                n203 = property on="Bottom Coil" class="Bool (strict)"("Val(Sgnl)"=w662) -> ()  [unwired: 2 in, 2 out]
                              }
                            }
                            n204 = local read "READY"() -> (w540:bool)
                            n205 = Not(x=w540) -> (.not. x?=w539:bool)
                            n206 = local read "Kill Switch"() -> (w543:bool)
                            n207 = Or(x=w544, y=w543) -> (x .or. y?=w542:bool)
                            n208 = Or(x=w539, y=w542) -> (x .or. y?=w541:bool)
                          }
                        }
                        frame #7 {
                          n209 = Decrement(x=w699) -> (x-1=w698:i32)
                          n210 = Equal?(x=w700, y=w698) -> (x = y?=w701:bool)
                          n211 = case shown="False" w701 {
                            tunnel: w689 -> [w710 w715]
                            tunnel: [w709 w722] -> w697
                            tunnel: w696 -> [w705 _]
                            tunnel: [w703 w716] -> w695
                            frame False {
                              w702 = FALSE ("Value (Signaling)")
                              n212 = Number To Decimal String(number=w710) -> (decimal integer string=w707:string)  [unwired: 1 in]
                              n213 = property on="Top Coil" class="Bool (strict)"("Val(Sgnl)"=w702) -> ()  [unwired: 2 in, 2 out]
                              n214 = property on="Bottom Coil" class="Bool (strict)"("Val(Sgnl)"=w702) -> ()  [unwired: 2 in, 2 out]
                              n215 = property on="SCRIPTING" class="Bool (strict)"("Val(Sgnl)"=w702) -> ()  [unwired: 2 in, 2 out]
                              n216 = property on="Neutron Shutter" class="Bool (strict)"("Val(Sgnl)"=w702) -> ()  [unwired: 2 in, 2 out]
                              n217 = property on="DATA" class="Bool (strict)"("Val(Sgnl)"=w702) -> ()  [unwired: 2 in, 2 out]
                              n218 = property on="RUN/STOP" class="Bool (strict)"("Val(Sgnl)"=w702) -> ()  [unwired: 2 in, 2 out]
                              n219 = Concatenate Strings("Script" ("string"), w707, " failed!" ("string"), "\r\n", w705) -> (w703:string)
                              n220 = Bundle(FALSE, 1017, w703) -> (w709:errorcluster)  [unwired: 1 in]
                              n221 = property on="Enable" class="Bool (strict)"("Val(Sgnl)"=w702) -> ()  [unwired: 2 in, 2 out]
                            }
                            frame True {
                              n222 = Number To Decimal String(number=w715) -> (decimal integer string=w718:string)  [unwired: 1 in]
                              n223 = Less?(x=w715, y="Script\nEnd") -> (x < y?=w713:bool)
                              n224 = case shown="True" w713 {
                                tunnel: w715 -> [_ w725]
                                frame False {
                                n225 = property on="SCRIPTING" class="Bool (strict)"("Val(Sgnl)"=FALSE ("Value (Signaling)")) -> ()  [unwired: 2 in, 2 out]
                                }
                                frame True {
                                n226 = Increment(x=w725) -> (x+1=w726:u32)
                                n227 = property on="Script\n#" class="DigNum (strict)"("Val(Sgnl)"=w726) -> ()  [unwired: 2 in, 2 out]
                                n228 = Wait (ms)(milliseconds to wait=u32 5000) -> ()  [unwired: 1 out]
                                }
                              }
                              n229 = Concatenate Strings("Script" ("string"), w718, " successful!" ("string")) -> (w716:string)
                              n230 = Bundle(FALSE, 0, w716) -> (w722:errorcluster)  [unwired: 1 in]
                            }
                          }
                          "Scripting \nError" <- w697
                          n231 = local read "Timestamp"() -> (w690:string)
                          n232 = call "WriteResults_Script.vi"("Timestamp"=w690, "error in"=w693, "Result"=w695, "refnum in"=w694) -> ("error out"=w691:errorcluster, "refnum out"=w692:refnum<file>)  [unwired: 6 in]
                        }
                      }
                      n233 = Array Size(array=w498) -> (size(s)=w497:i32)
                    }
                  }
                  n234 = flat-sequence {
                    tunnel: w455 -> [w465]
                    tunnel: [w465] -> w454
                    tunnel: [w464] -> w453
                    frame #0 {
                      n235 = local read "READY"() -> (w468:bool)
                      n236 = local read "SCRIPTING"() -> (w470:bool)
                      n237 = local read "Kill Switch"() -> (w467:bool)
                      n238 = Not(x=w468) -> (.not. x?=w469:bool)
                      n239 = Or(x=w469, y=w467) -> (x .or. y?=w466:bool)
                      n240 = Not(x=w470) -> (.not. x?=w471:bool)
                      n241 = Or(x=w471, y=w466) -> (x .or. y?=w464:bool)
                    }
                  }
                }
              }
            }
          }
        }
      }
      event Timeout {
        n242 = event-data() -> ()  [unwired: 1 in, 3 out]
      }
    }
    n243 = local read "Kill Switch"() -> (w243:bool)
  }
  n244 = while {
    shift-right: [w750] -> _
    shift-left: _ -> [w748]
    shift-right: [w751] -> _
    shift-left: _ -> [w749]
    shift-right: [w744] -> w49
    shift-left: w121 -> [w746]
    shift-right: [w745] -> w50
    shift-left: w120 -> [w747]
    shift-right: [w740] -> w54
    shift-left: w95 -> [w743]
    shift-right: [w741] -> w52
    shift-left: w93 -> [w742]
    shift-right: [w735] -> w99
    shift-left: w56 -> [w738]
    shift-right: [w736] -> w100
    shift-left: w55 -> [w737]
    shift-right: [w730] -> w16
    shift-left: w19 -> [w732]
    shift-right: [w729] -> w15
    shift-left: w18 -> [w731]
    stop <- "Kill Switch" stop-if-true
    n245 = event shown="[5] \"On CCD Accumulations\", \"Number of Frames\": Value Change" {
      selector: _ -> [_ _ _ _ _ _ _ _ _]
      dyn-events: _ -> [_ _ _ _ _ _ _ _ _]
      timeout: 500 -> [_ _ _ _ _ _ _ _ _]
      tunnel: w747 -> [w759 w768 w816 w840 w868 w907 w932 w943 w956]
      tunnel: w746 -> [w758 w767 w817 w841 w867 w908 w933 w942 w955]
      tunnel: w749 -> [w760 w771 w809 w837 w871 w913 w930 w946 w960]
      tunnel: w748 -> [w761 w772 w810 w836 w872 w914 w931 w947 w959]
      tunnel: [w760 w773 w809 w834 w871 w911 w930 w946 w960] -> w751
      tunnel: [w761 w774 w810 w835 w872 w912 w931 w947 w959] -> w750
      tunnel: [w759 w768 w819 w840 w868 w904 w932 w943 w956] -> w745
      tunnel: [w758 w767 w818 w841 w867 w903 w933 w942 w955] -> w744
      tunnel: w743 -> [w756 w769 w813 w838 w874 w906 w939 w945 w958]
      tunnel: w742 -> [w757 w770 w814 w839 w873 w905 w938 w944 w957]
      tunnel: [w757 w770 w814 w839 w873 w905 w935 w944 w957] -> w741
      tunnel: [w756 w769 w813 w838 w874 w906 w934 w945 w958] -> w740
      tunnel: w738 -> [w755 w766 w812 w842 w870 w910 w929 w941 w954]
      tunnel: w737 -> [w754 w765 w811 w843 w869 w909 w928 w940 w953]
      tunnel: [w754 w765 w811 w843 w866 w909 w928 w940 w953] -> w736
      tunnel: [w755 w766 w812 w842 w865 w910 w929 w941 w954] -> w735
      tunnel: "LIGHTFIELD" -> [_ _ _ w833 _ w902 _ _ _]
      tunnel: w732 -> [w752 w763 w808 w831 w863 w901 w926 w951 w964]
      tunnel: w731 -> [w753 w762 w807 w830 w862 w900 w925 w950 w963]
      tunnel: [w752 w763 w808 w831 w863 w901 w926 w949 w961] -> w730
      tunnel: [w753 w762 w807 w830 w862 w900 w925 w948 w962] -> w729
      event Timeout {
        n246 = event-data() -> ()  [unwired: 1 in, 3 out]
      }
      event "LIGHTFIELD": Value Change {
        n247 = event-data() -> ("NewVal"=w764:bool)  [unwired: 1 in, 5 out]
        n248 = case shown="True" w764 {
          tunnel: [refnum<class "LightField Automation.lvclass"> refnum ("LightField Automation out") w786] -> w774
          tunnel: [errorcluster {"status"=FALSE, "code"=0, "source"=""} ("error out") w785] -> w773
          tunnel: w772 -> [w778 _]
          tunnel: w771 -> [w777 _]
          frame False {
            n249 = call "Adv_Deregister_for_Callback.vi"("error in (no error)"=w777, "LightField Automation in"=w778) -> ("error out"=w780:errorcluster, "LightField Automation out"=w781:refnum<class "LightField Automation.lvclass">)  [unwired: 8 in]
            n250 = call "LFA_Close.vi"("error in (no error)"=w780, "LightField Automation in"=w781) -> ("error out"=→"LightField Error":errorcluster)  [unwired: 8 in, 1 out]
          }
          frame True {
            n251 = call "LFA_Initialize.vi"("error in (no error)"=errorcluster {"status"=FALSE, "code"=0, "source"=""}) -> ("error out"=w796:errorcluster, "LightField Automation out"=w795:refnum<class "LightField Automation.lvclass">)  [unwired: 9 in]
            n252 = call "Adv_Register_for_Callback.vi"("error in (no error)"=w796, "LightField Automation in"=w795) -> ("error out"=w794:errorcluster, "LightField Automation out"=w793:refnum<class "LightField Automation.lvclass">)  [unwired: 8 in]
            n253 = call "Exp_SetExperiment.vi"("error in (no error)"=w794, "ExperimentName"="Experiment1", "LightField Automation in"=w793) -> ("error out"=w799:errorcluster, "LightField Automation out"=w798:refnum<class "LightField Automation.lvclass">)  [unwired: 7 in]
            n254 = Multiply(x=0.25, y=1000.0) -> (x*y=w806:dbl)
            n255 = Multiply(x=10.0, y=1000.0) -> (x*y=w797:dbl)
            n256 = local read "On CCD Accumulations"() -> (w787:i32)
            n257 = call "Exp_ICCD_SetRepetitiveGateProperties.vi"("error in (no error)"=w799, "Repetitive Gate Width (ns)"=w797, "Repetitive Gate Delay (ns)"=w806, "LightField Automation in"=w798) -> ("error out"=w800:errorcluster, "LightField Automation out"=w801:refnum<class "LightField Automation.lvclass">)  [unwired: 6 in]
            n258 = local read "Number of Frames"() -> (w788:i32)
            n259 = call "Exp_ICCD_SetIntensifierGain.vi"("error in (no error)"=w800, "Intensifier Gain"=100, "LightField Automation in"=w801) -> ("error out"=w802:errorcluster, "LightField Automation out"=w803:refnum<class "LightField Automation.lvclass">)  [unwired: 7 in]
            n260 = call "Exp_SetFrames.vi"("error in (no error)"=w802, "Number of Frames"=w788, "LightField Automation in"=w803) -> ("error out"=w805:errorcluster, "LightField Automation out"=w804:refnum<class "LightField Automation.lvclass">)  [unwired: 7 in]
            n261 = call "Exp_ICCD_SetOnChipAccumulations.vi"("error in (no error)"=w805, "On Chip Accumulations"=w787, "LightField Automation in"=w804) -> ("error out"=w785:errorcluster, "LightField Automation out"=w786:refnum<class "LightField Automation.lvclass">)  [unwired: 7 in]
          }
        }
      }
      event "RUN/STOP": Value Change {
        n262 = event-data() -> ("NewVal"=w815:bool)  [unwired: 1 in, 5 out]
        n263 = case shown="False" w815 {
          tunnel: [w821 w829] -> w819
          tunnel: [w822 w828] -> w818
          tunnel: w817 -> [w823 w827]
          tunnel: w816 -> [w824 w826]
          frame False {
            n264 = VISA Write(VISA resource name=w823, write buffer=":PULSE0:STATE OFF\r\n" ("format string"), error in (no error)=w824) -> (VISA resource name out=w822:refnum<visa-resource-name>, error out=w821:errorcluster)  [unwired: 1 out]
          }
          frame True {
            n265 = VISA Write(VISA resource name=w827, write buffer=":PULSE0:STATE ON\r\n" ("format string"), error in (no error)=w826) -> (VISA resource name out=w828:refnum<visa-resource-name>, error out=w829:errorcluster)  [unwired: 1 out]
          }
        }
      }
      event "DATA": Value Change {
        n266 = event-data() -> ("NewVal"=w832:bool)  [unwired: 1 in, 5 out]
        n267 = case shown="True" w832 {
          tunnel: w837 -> [w844 w849]
          tunnel: w836 -> [w845 w850]
          tunnel: [w845 w848] -> w835
          tunnel: [w844 w847] -> w834
          tunnel: w833 -> [_ w851]
          frame False {
            n268 = local write "CLOSE"(TRUE ("CLOSE")) -> ()
          }
          frame True {
            n269 = case shown="True" w851 {
              tunnel: w849 -> [w853 w858]
              tunnel: w850 -> [w854 w857]
              tunnel: [w854 w856] -> w848
              tunnel: [w853 w855] -> w847
              frame False {
              }
              frame True {
                n270 = call "LFA_AcquireWithAutosave.vi"("error in (no error)"=w858, "LightField Automation in"=w857) -> ("error out"=w855:errorcluster, "LightField Automation out"=w856:refnum<class "LightField Automation.lvclass">)  [unwired: 7 in, 1 out]
              }
            }
            n271 = local write "RECORD"(TRUE ("RECORD")) -> ()
          }
        }
      }
      event "Percent Open": Value Change {
        n272 = event-data() -> ("OldVal"=w864:i32, "NewVal"=w875:i32)  [unwired: 1 in, 4 out]
        n273 = Subtract(x=w875, y=w864) -> (x-y=w859:i32)
        n274 = Greater Than 0?(x=w859) -> (x > 0?=w860:bool)
        n275 = Equal To 0?(x=w875) -> (x = 0?=w861:bool)
        n276 = case shown="False" w861 {
          tunnel: w869 -> [w879 w895]
          tunnel: w870 -> [w880 w894]
          tunnel: [w878 w893] -> w866
          tunnel: [w877 w892] -> w865
          tunnel: w860 -> [w881 _]
          tunnel: w859 -> [w876 _]
          frame False {
            n277 = case shown="False" w881 {
              tunnel: w880 -> [w885 w891]
              tunnel: w879 -> [w886 w890]
              tunnel: [w884 w889] -> w878
              tunnel: [w883 w888] -> w877
              tunnel: w876 -> [w882 w887]
              frame False {
                n278 = call "NeedleValveClose - Encoder.vi"("error in (no error)"=w885, "Percent Difference"=w882, "VISA resource name"=w886) -> ("error out"=w883:errorcluster, "VISA resource name out"=w884:refnum<visa-resource-name>)  [unwired: 7 in]
              }
              frame True {
                n279 = call "NeedleValveOpen - Encoder.vi"("error in (no error)"=w891, "Percent Difference"=w887, "VISA resource name"=w890) -> ("error out"=w888:errorcluster, "VISA resource name out"=w889:refnum<visa-resource-name>)  [unwired: 7 in]
              }
            }
          }
          frame True {
            n280 = call "NeedleValveClose.vi"("error in (no error)"=w894, "VISA resource name"=w895) -> ("error out"=w892:errorcluster, "VISA resource name out"=w893:refnum<visa-resource-name>)  [unwired: 8 in]
          }
        }
      }
      event "On CCD Accumulations", "Number of Frames": Value Change {
        n281 = event-data() -> ()  [unwired: 1 in, 4 out]
        n282 = call "PGIntialize.vi"("On CCD Accumulations"="On CCD Accumulations", "Number of Frames"="Number of Frames", "error in"=w907, "BIN"="BIN", "MODE"="MODE", "VISA resource name"=w908) -> ("error out"=w904:errorcluster, "VISA resource name out"=w903:refnum<visa-resource-name>)  [unwired: 4 in]
        n283 = case shown="True" w902 {
          tunnel: w914 -> [w915 w924]
          tunnel: w913 -> [w916 w923]
          tunnel: [w915 w920] -> w912
          tunnel: [w916 w919] -> w911
          tunnel: "On CCD Accumulations" -> [_ w918]
          tunnel: "Number of Frames" -> [_ w917]
          frame False {
          }
          frame True {
            n284 = call "Exp_SetFrames.vi"("error in (no error)"=w923, "Number of Frames"=w917, "LightField Automation in"=w924) -> ("error out"=w921:errorcluster, "LightField Automation out"=w922:refnum<class "LightField Automation.lvclass">)  [unwired: 7 in]
            n285 = call "Exp_ICCD_SetOnChipAccumulations.vi"("error in (no error)"=w921, "On Chip Accumulations"=w918, "LightField Automation in"=w922) -> ("error out"=w919:errorcluster, "LightField Automation out"=w920:refnum<class "LightField Automation.lvclass">)  [unwired: 7 in]
          }
        }
      }
      event "Siphon Pump", "Sample Space Pump", "Neutron Shutter": Value Change {
        n286 = event-data() -> ()  [unwired: 1 in, 6 out]
        n287 = call "RelayControl.vi"("Neutron Shutter"="Neutron Shutter", "Error In"=w939, "Sample Space Pump"="Sample Space Pump", "Siphon Pump"="Siphon Pump", "Relay In"=w938) -> ("Error Out"=w934:errorcluster, "Relay Out"=w935:refnum<visa-resource-name>)  [unwired: 5 in]
      }
      event "Enable": Value Change {
        n288 = event-data() -> ()  [unwired: 1 in, 6 out]
        n289 = call "ToggleShutter.vi"("error in"=w950, "VISA resource name"=w951) -> ("error out"=w948:errorcluster, "VISA resource name out"=w949:refnum<visa-resource-name>)  [unwired: 8 in]
      }
      event "Shutter Mode": Value Change {
        n290 = event-data() -> ("NewVal"=w952:u16)  [unwired: 1 in, 5 out]
        n291 = call "ThorlabsMode.vi"("error in"=w963, "Mode"=w952, "VISA resource name"=w964) -> ("error out"=w962:errorcluster, "VISA resource name out"=w961:refnum<visa-resource-name>)  [unwired: 7 in]
      }
    }
  }
  n292 = while {
    shift-right: [w1030] -> w113
    shift-left: w112 -> [w1029]
    shift-right: [w1031] -> w114
    shift-left: w111 -> [w1028]
    shift-right: [w1025] -> w104
    shift-left: w109 -> [w1027]
    shift-right: [w1024] -> w103
    shift-left: w108 -> [w1026]
    shift-right: [w1023] -> w35
    shift-left: _ -> [w1021]
    shift-right: [w1022] -> w34
    shift-left: _ -> [w1020]
    shift-right: [w1017] -> w59
    shift-left: w72 -> [w1019]
    shift-right: [w1016] -> w61
    shift-left: w73 -> [w1015]
    shift-right: [w1013] -> w76
    shift-left: w98 -> [w1014]
    shift-right: [w1011] -> w77
    shift-left: w97 -> [w1012]
    tunnel: w74 -> [w1018]
    tunnel: [w982] -> w60
    shift-right: [w979] -> w39
    shift-left: w41 -> [w981]
    shift-right: [w978] -> w38
    shift-left: w40 -> [w980]
    shift-right: [w971] -> _
    shift-left: _ -> [w970]
    stop <- w972 stop-if-true
    n293 = local read "DATA"() -> (w977:bool)
    n294 = call "Collect Data.vi"("Location of FieldMax2Lib.dll in"=w980, "Meter ID in"=w981) -> ("Location of FieldMax2Lib.dll out"=w978:path, "Meter ID out"=w979:i32, "Measurement"=w975:sgl)  [unwired: 5 in, 1 out]
    n295 = Multiply(x="Data Interval (s)", y=u32 1000 ("millisecond multiple")) -> (x*y=w983:dbl)
    n296 = Multiply(x=w975, y=1000.0) -> (x*y=w974:dbl)
    "Power (mW)" <- w974
    n297 = Get Date/Time String(want seconds? (F)=TRUE) -> (time string=→"time string":string)  [unwired: 2 in, 1 out]
    n298 = case shown="True" "RECORD" {
      tunnel: w1021 -> [w1082 _]
      tunnel: w1020 -> [w1083 _]
      tunnel: [w1083 w1088] -> w986
      tunnel: [w1082 w1087] -> w988
      frame False {
      }
      frame True {
        n299 = local read "SCRIPTING"() -> (w1086:bool)
        n300 = local read "Script\n#"() -> (w1085:u32)
        n301 = local write "RECORD"(FALSE ("RECORD")) -> ()
        n302 = call "DataHeader.vi"("Script #"=w1085, "Scripting"=w1086) -> ("error out"=w1087:errorcluster, "Timestamp"=→"Timestamp":string, "refnum out"=w1088:refnum<file>)  [unwired: 7 in]
      }
    }
    n303 = call-poly "Open.vi"("error in (no error)"=w1028, "Device Identifier"="MB1.T1:TEMP", "Mercury Reference In"=w1029) -> ("error out"=w1003:errorcluster, "Mercury Reference Out"=w1002:T4)  [unwired: 7 in]
    n304 = call-poly "Signals (Read).vi"("error in"=w1003, "Mercury Reference In"=w1002) -> ("error out"=w1000:errorcluster, "Temperature"=w989:dbl, "Mercury Reference Out"=w1001:T4)  [unwired: 5 in, 2 out]
    "Cryostat Temp (K)" <- w989
    n305 = call-poly "Open.vi"("error in (no error)"=w1000, "Device Identifier"="DB6.T1:TEMP", "Mercury Reference In"=w1001) -> ("error out"=w998:errorcluster, "Mercury Reference Out"=w999:T4)  [unwired: 7 in]
    n306 = call "PressureControl - 3He.vi"("error in (no error)"=w1014, "VISA resource name"=w1012) -> ("error out"=w1013:errorcluster, "3HePressure (Torr)"=w991:string, "VISA resource name out"=w1011:refnum<visa-resource-name>)  [unwired: 7 in]
    n307 = call "PressureControl - 4He.vi"("error in (no error)"=w1027, "VISA resource name"=w1026) -> ("error out"=w1025:errorcluster, "Pressure"=w993:dbl, "Pressure (Torr)"=w987:string, "VISA resource name out"=w1024:refnum<visa-resource-name>)  [unwired: 6 in]
    n308 = call-poly "Signals (Read).vi"("error in"=w998, "Mercury Reference In"=w999) -> ("error out"=w1031:errorcluster, "Temperature"=w990:dbl, "Mercury Reference Out"=w1030:T4)  [unwired: 5 in, 2 out]
    "Cell Temp (K)" <- w990
    n309 = case shown="\"Main Controls\", Default" "Turbulence" {
      tunnel: w987 -> [w1090 w1094]
      tunnel: w991 -> [w1091 w1093]
      tunnel: "Log Pressure" -> [_ w1092]
      frame "Main Controls", Default {
        "Tank Pressure 2 (Torr)" <- w1091
        "Tank Pressure 1 (Torr)" <- w1090
      }
      frame "Fill Tanks" {
        n310 = call "SaveTankData.vi"("Log Pressure"=w1092, "4He Pressure (Torr)"=w1094, "3He Pressure (Torr)"=w1093) -> ()  [unwired: 8 in]
        "3He Pressure (Torr)" <- w1093
        "4He Pressure (Torr)" <- w1094
      }
    }
    n311 = Less?(x=w993, y=30.0) -> (x < y?=w992:bool)
    n312 = disable-structure shown="Disabled" {
      disable-tunnel: w992 -> [w1035 _]
      frame Disabled {
        n313 = case shown="True" w1035 {
          tunnel: [FALSE ("RUN/STOP") TRUE ("RUN/STOP")] -> w1032
          frame False {
          }
          frame True {
          }
        }
        n314 = property on="READY" class="Bool (strict)"() -> ("Value"=w1034:bool)  [unwired: 2 in, 2 out]
        n315 = Equal?(x=w1034, y=w1032) -> (x = y?=w1033:bool)
        n316 = case shown="False" w1033 {
          tunnel: w1032 -> [w1036 _]
          frame False {
            n317 = property on="READY" class="Bool (strict)"("Val(Sgnl)"=w1036) -> ()  [unwired: 2 in, 2 out]
          }
          frame True {
          }
        }
      }
      frame Enabled {
      }
    }
    n318 = local read "Kill Switch"() -> (w972:bool)
    n319 = call "DAQ Assistant"("stop (F)"=w972) -> ("data"=w971:dynamicdata)  [unwired: 15 in, 3 out]
    "Neutron Counts" <- w971
    n320 = case shown="True" w977 {
      tunnel: w1015 -> [w1042 w1071]
      tunnel: w1019 -> [w1044 w1070]
      tunnel: w1018 -> [w1043 w1069]
      tunnel: [w1043 w1065] -> w997
      tunnel: [w1042 w1064] -> w996
      tunnel: [w1044 w1063] -> w995
      tunnel: w990 -> [_ w1057]
      tunnel: w989 -> [_ w1055]
      tunnel: w988 -> [w1040 w1054]
      tunnel: w987 -> [_ w1053]
      tunnel: w986 -> [w1041 w1052]
      tunnel: [w1040 w1051] -> w985
      tunnel: [w1041 w1050] -> w984
      tunnel: w983 -> [w1039 w1048]
      tunnel: [w1039 w1047] -> w973
      tunnel: w974 -> [_ w1046]
      tunnel: w971 -> [_ w1045]
      frame False {
      }
      frame True {
        n321 = Subtract(x=w1048, y=350.0) -> (x-y=w1047:dbl)
        n322 = call "Measure.vi"("Function (Current)"=T6."Power", "error in (no error)"=w1071, "Node In"=w1069, "VISA resource name"=w1070) -> ("error out"=w1062:errorcluster, "Output"=w1056:string, "Node Out"=w1066:string, "VISA resource name out"=w1067:refnum<visa-resource-name>)  [unwired: 3 in, 1 out]
        n323 = flat-sequence {
          tunnel: w1062 -> [w1072]
          tunnel: [w1072] -> w1061
          frame #0 {
            n324 = Wait (ms)(milliseconds to wait=u32 100) -> ()  [unwired: 1 out]
          }
        }
        n325 = call "Measure.vi"("Function (Current)"=T6."Power", "error in (no error)"=w1061, "Channel (Channel A)"=Channel."Channel B", "Node In"=w1066, "VISA resource name"=w1067) -> ("error out"=w1064:errorcluster, "Output"=w1058:string, "Node Out"=w1065:string, "VISA resource name out"=w1063:refnum<visa-resource-name>)  [unwired: 2 in, 1 out]
        n326 = call "CompileData.vi"("Detected"=w1045, "Ch. B (W)"=w1058, "Cell Temp (K)"=w1057, "Ch. A (W)"=w1056, "Cryostat Temp (K)"=w1055, "error in"=w1054, "Laser Power (W)"=w1046, "Tank Pressure (Torr)"=w1053, "refnum in"=w1052) -> ("error out"=w1051:errorcluster, "refnum out"=w1050:refnum<file>)  [unwired: 1 in]
      }
    }
    n327 = case shown="True" "CLOSE" {
      tunnel: w985 -> [w1074 w1080]
      tunnel: w984 -> [w1075 w1079]
      tunnel: [w1075 refnum<file> refnum ("refnum out")] -> w1022
      tunnel: [w1074 errorcluster {"status"=FALSE, "code"=0, "source"=""} ("error out")] -> w1023
      frame False {
      }
      frame True {
        n328 = local write "CLOSE"(FALSE ("CLOSE")) -> ()
        n329 = Close File(refnum=w1079, error in=w1080) -> (error out=→"File I/O Error":errorcluster)  [unwired: 1 out]
      }
    }
    n330 = event shown="[4] \"Bottom Coil\": Value Change" {
      selector: _ -> [_ _ _ _ _]
      dyn-events: _ -> [_ _ _ _ _]
      timeout: w973 -> [_ _ _ _ _]
      tunnel: w997 -> [w1095 w1105 w1113 w1121 w1129]
      tunnel: w996 -> [w1096 w1106 w1115 w1123 w1131]
      tunnel: w995 -> [w1097 w1104 w1112 w1120 w1128]
      tunnel: [w1097 w1103 w1114 w1122 w1130] -> w1017
      tunnel: [w1096 w1099 w1108 w1118 w1125] -> w1016
      tunnel: [w1095 w1098 w1107 w1117 w1124] -> w982
      event Timeout {
        n331 = event-data() -> ()  [unwired: 1 in, 3 out]
      }
      event "Top Coil (mA)": Value Change {
        n332 = event-data() -> ("NewVal"=w1101:dbl)  [unwired: 1 in, 5 out]
        n333 = Divide(x=w1101, y=1000.0) -> (x/y=w1100:dbl)
        n334 = call "Source Level.vi"("Level (0.000)"=w1100, "error in (no error)"=w1106, "Node In"=w1105, "VISA resource name"=w1104) -> ("error out"=w1099:errorcluster, "Node Out"=w1098:string, "VISA resource name out"=w1103:refnum<visa-resource-name>)  [unwired: 4 in, 1 out]
      }
      event "Bottom Coil (mA)": Value Change {
        n335 = event-data() -> ("NewVal"=w1110:dbl)  [unwired: 1 in, 5 out]
        n336 = Divide(x=w1110, y=1000.0) -> (x/y=w1109:dbl)
        n337 = call "Source Level.vi"("Level (0.000)"=w1109, "error in (no error)"=w1115, "Channel (Channel A)"=Channel."Channel B", "Node In"=w1113, "VISA resource name"=w1112) -> ("error out"=w1108:errorcluster, "Node Out"=w1107:string, "VISA resource name out"=w1114:refnum<visa-resource-name>)  [unwired: 3 in, 1 out]
      }
      event "Top Coil": Value Change {
        n338 = event-data() -> ("NewVal"=w1119:bool)  [unwired: 1 in, 5 out]
        n339 = call "Source Output Enable.vi"("Output (Off)"=w1119, "error in (no error)"=w1123, "Node In"=w1121, "VISA resource name"=w1120) -> ("error out"=w1118:errorcluster, "Node Out"=w1117:string, "VISA resource name out"=w1122:refnum<visa-resource-name>)  [unwired: 4 in, 1 out]
      }
      event "Bottom Coil": Value Change {
        n340 = event-data() -> ("NewVal"=w1126:bool)  [unwired: 1 in, 5 out]
        n341 = call "Source Output Enable.vi"("Output (Off)"=w1126, "error in (no error)"=w1131, "Channel (Channel A)"=Channel."Channel B", "Node In"=w1129, "VISA resource name"=w1128) -> ("error out"=w1125:errorcluster, "Node Out"=w1124:string, "VISA resource name out"=w1130:refnum<visa-resource-name>)  [unwired: 3 in, 1 out]
      }
    }
    n342 = Subtract(1:w970, 2:w971) -> (0:w968:dynamicdata)  [unwired: 1 in, 1 out]
    n343 = Divide(x=w968, y="Data Interval (s)") -> (x/y=→"Rate (Hz)":dynamicdata)
  }
  n344 = call "NeedleValveClose.vi"("error in (no error)"=w99, "VISA resource name"=w100) -> ("error out"=w6:errorcluster, "VISA resource name out"=w8:refnum<visa-resource-name>)  [unwired: 8 in]
  n345 = VISA Close(VISA resource name=w16, error in (no error)=w15) -> ()  [unwired: 1 out]
  n346 = call "RelayControl.vi"("Neutron Shutter"=w33, "Error In"=w54, "Sample Space Pump"=w33, "Siphon Pump"=w33, "Relay In"=w52) -> ("Error Out"=w53:errorcluster, "Relay Out"=w51:refnum<visa-resource-name>)  [unwired: 5 in]
  n347 = flat-sequence {
    tunnel: [w1135] -> w47
    tunnel: [w1134] -> w48
    tunnel: w49 -> [w1133]
    tunnel: w50 -> [w1132]
    frame #0 {
      n348 = VISA Write(VISA resource name=w1133, write buffer=":PULSE0:STATE OFF\r\n" ("format string"), error in (no error)=w1132) -> (VISA resource name out=w1134:refnum<visa-resource-name>, error out=w1135:errorcluster)  [unwired: 1 out]
    }
  }
  n349 = VISA Close(VISA resource name=w51, error in (no error)=w53) -> (error out=w46:errorcluster)
  n350 = flat-sequence {
    tunnel: w6 -> [w1137]
    tunnel: [w1137] -> w9
    tunnel: [w1140] -> w7
    tunnel: w9 -> [w1140]
    frame #0 {
      n351 = Wait (ms)(milliseconds to wait=u32 3000) -> ()  [unwired: 1 out]
    }
    frame #1 {
      n352 = local write "Percent Open"(0 ("Percent Open")) -> ()
    }
  }
  n353 = flat-sequence {
    tunnel: w33 -> [w1141]
    tunnel: [w1142] -> w45
    tunnel: w46 -> [w1142]
    frame #0 {
      n354 = local write "Siphon Pump"(w1141) -> ()
      n355 = local write "Sample Space Pump"(w1141) -> ()
      n356 = local write "Neutron Shutter"(w1141) -> ()
    }
  }
  n357 = call "Close.vi"("error in (no error)"=w114, "Mercury Reference"=w113) -> ("error out"=w67:errorcluster)  [unwired: 9 in]
  n358 = call "Disconnect From Meter.vi"("Location of FieldMax2Lib.dll in"=w38, "Meter ID in"=w39) -> ()  [unwired: 7 in, 2 out]
  n359 = call "KeithleyClose.vi"("Keithley Error In"=w61, "Node In"=w60, "KeithleyVISA In"=w59) -> ("Heater Error"=w58:errorcluster)  [unwired: 8 in]
  n360 = VISA Close(VISA resource name=w103, error in (no error)=w104) -> (error out=→"4He Gauge Error":errorcluster)
  n361 = call "3HeClose.vi"("error in (no error)"=w76, "VISA resource name"=w77) -> ("error out"=→"3He Gauge Error":errorcluster)  [unwired: 9 in]
  n362 = Not Equal?(x=refnum<file> refnum, y=w34) -> (x != y?=w36:bool)
  n363 = VISA Close(VISA resource name=w48, error in (no error)=w47) -> (error out=→"Pulse Generator Error":errorcluster)
  n364 = flat-sequence {
    tunnel: w58 -> [w1144]
    tunnel: [w1144] -> w57
    frame #0 {
      w1143 = FALSE ("Top Coil")
      n365 = local write "Top Coil"(w1143) -> ()
      n366 = local write "Bottom Coil"(w1143) -> ()
    }
  }
  n367 = VISA Close(VISA resource name=w8, error in (no error)=w7) -> (error out=w65:errorcluster)
  n368 = case shown="True" w36 {
    tunnel: w35 -> [_ w1147]
    tunnel: w34 -> [_ w1146]
    frame False {
    }
    frame True {
      n369 = Close File(refnum=w1146, error in=w1147) -> (error out=w1145:errorcluster)  [unwired: 1 out]
      n370 = local write "File I/O Error"(w1145) -> ()
    }
  }
  n371 = flat-sequence {
    tunnel: w67 -> [w1153]
    tunnel: [w1153] -> w66
    tunnel: w65 -> [w1152]
    tunnel: [w1152] -> w64
    tunnel: w63 -> [w1151]
    tunnel: [w1151] -> w62
    tunnel: [T2 {"status"=FALSE, "code"=0, "Description"=""} ("Scripting \nError")] -> w32
    tunnel: [w1148] -> w25
    tunnel: w26 -> [w1148]
    frame #0 {
      w1150 = FALSE ("Kill Switch")
      n372 = local write "Kill Switch"(w1150) -> ()
      n373 = local write "READY"(w1150) -> ()
    }
  }
  n374 = local write "Scripting \nError"(w32) -> ()
  n375 = TCP Close Connection(connection ID=w85, error in (no error)=w86) -> (error out=w63:errorcluster)  [unwired: 1 in, 1 out]
  n376 = Close File(refnum=w28, error in=w27) -> (error out=w26:errorcluster)  [unwired: 1 out]
  "Temperature Error" <- w66
  "Heater Error" <- w57
  "Relay Errror" <- w45
  "Zaber Motor Error" <- w64
  "Level Probe Error" <- w62
  "Log Error" <- w25
